vi "value to ring (PayloadBufferMode).vi"(11 "value":string) -> (3 "PayloadBufferMode":i32)   [LabVIEW 2020, in "AIM ARINC 664 Import.lvlib"]
uses:
  AIM ARINC 664 Import.lvlib
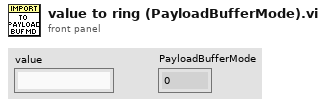
[diagram p1: front panel]
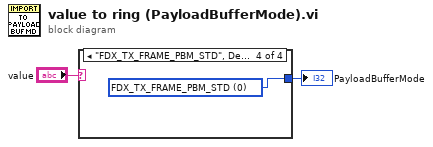
[diagram p0: block diagram]
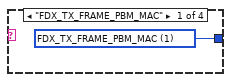
[diagram p2: hidden frame]
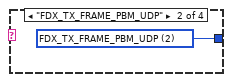
[diagram p3: hidden frame]
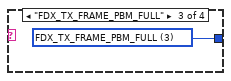
[diagram p4: hidden frame]
diagram:
  n1 = case shown="\"FDX_TX_FRAME_PBM_STD\", Default" "value" {
    tunnel: [w3 w4 w5 w6] -> w1
    frame "FDX_TX_FRAME_PBM_MAC" {
      w3 = 1 items=["FDX_TX_FRAME_PBM_STD", "FDX_TX_FRAME_PBM_MAC", "FDX_TX_FRAME_PBM_UDP", "FDX_TX_FRAME_PBM_FULL"] ("PayloadBufferMode")
    }
    frame "FDX_TX_FRAME_PBM_UDP" {
      w4 = 2 items=["FDX_TX_FRAME_PBM_STD", "FDX_TX_FRAME_PBM_MAC", "FDX_TX_FRAME_PBM_UDP", "FDX_TX_FRAME_PBM_FULL"] ("PayloadBufferMode")
    }
    frame "FDX_TX_FRAME_PBM_FULL" {
      w5 = 3 items=["FDX_TX_FRAME_PBM_STD", "FDX_TX_FRAME_PBM_MAC", "FDX_TX_FRAME_PBM_UDP", "FDX_TX_FRAME_PBM_FULL"] ("PayloadBufferMode")
    }
    frame "FDX_TX_FRAME_PBM_STD", Default {
      w6 = 0 items=["FDX_TX_FRAME_PBM_STD", "FDX_TX_FRAME_PBM_MAC", "FDX_TX_FRAME_PBM_UDP", "FDX_TX_FRAME_PBM_FULL"] ("PayloadBufferMode")
    }
  }
  "PayloadBufferMode" <- w1
